vi "Destroy User Event - Stop.vi"(8 "error in (no error)":errorcluster, 11 "User Event Bundle":T1) -> (0 "error out":errorcluster)   [LabVIEW 2018, in "User Event - Stop.lvlib"]
doc: "Destroy the user event, even if there is an incoming error."
uses:
  User Event - Stop.lvlib
  Type Defs/User Events.ctl
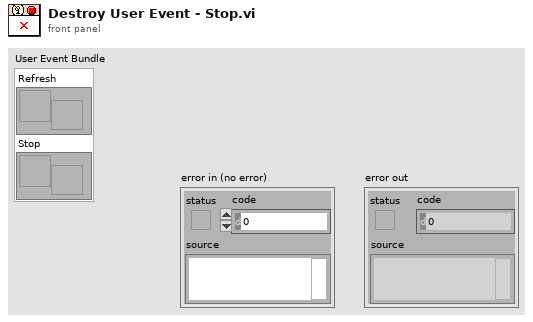
[diagram p1: front panel]
types:
  T1 = typedef "User Events.ctl" = cluster{"Refresh":refnum<user-event>, "Stop":refnum<user-event>}
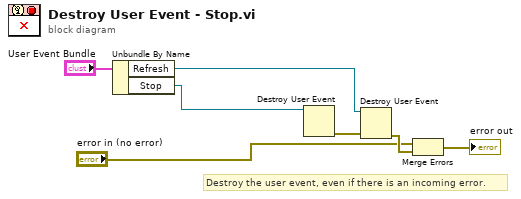
[diagram p0: block diagram]
diagram:
  # "Destroy the user event, even if there is an incoming error."
  n1 = Unbundle By Name("User Event Bundle") -> ("Refresh"=w1:refnum<user-event>, "Stop"=w2:refnum<user-event>)
  n2 = Destroy User Event(user event=w2) -> (error out=w3:errorcluster)  [unwired: 1 in]
  n3 = Destroy User Event(user event=w1, error in=w3) -> (error out=w7:errorcluster)
  n4 = Merge Errors("error in (no error)", w7) -> (→"error out":errorcluster)
